vi "Core.vi"(8 "error in (no error)":errorcluster, 11 "TCP in":refnum<class "TCP.lvclass">) -> (0 "error out":errorcluster, 3 "TCP out":refnum<class "TCP.lvclass">)   [LabVIEW 2021, in "TCP.lvclass"]
uses:
  TCP.lvclass
  D:/my_projects/projects/Algorithms/Labview/21/Modbus_v121c/Network Protocol/MB/Modbus Master CR.lvclass
  MB/ctl/MB_TCP_State.ctl
  MB/Modbus Master CR.lvclass/Modbus Master CR.ctl
  MB/Status/Run/Write Run.vi
  MB/Status/write/Write write.vi
  Data Model/Device Data Model.lvclass
  MB/Modbus Master CR.lvclass
panel:
  out "MB_TCP_State":T1=enum."requests"
  in  "write enable":bool=TRUE
  in  "stop":bool
  out "stopped":bool
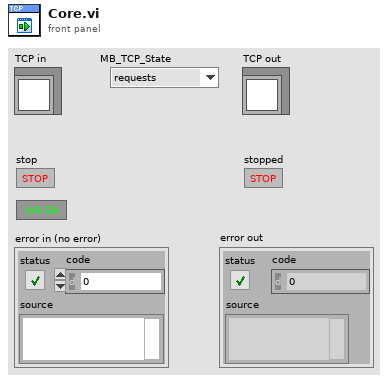
[diagram p1: front panel]
types:
  T1 = typedef "Modbus Master CR.lvclass/MB_TCP_State.ctl" = enum8{"initialization", "redefine", "standby", "ping", "connect", "wait to reconnect", "wait to reset timeout", "configure", "requests", "close connection", "stop"}
  T2 = typedef "Modbus Master CR.lvclass/MB timeouts.ctl" = cluster{"reconn_timeout":i32, "N attempt max":i32, "t_reset_TTL":i32, "period":i32}
  T3 = typedef "Modbus Master CR.lvclass/MB state.ctl" = cluster{"state":T1, "enable":bool, "Run":bool, "write enable":bool, "Write":bool, "connect":bool, "errors":i32}
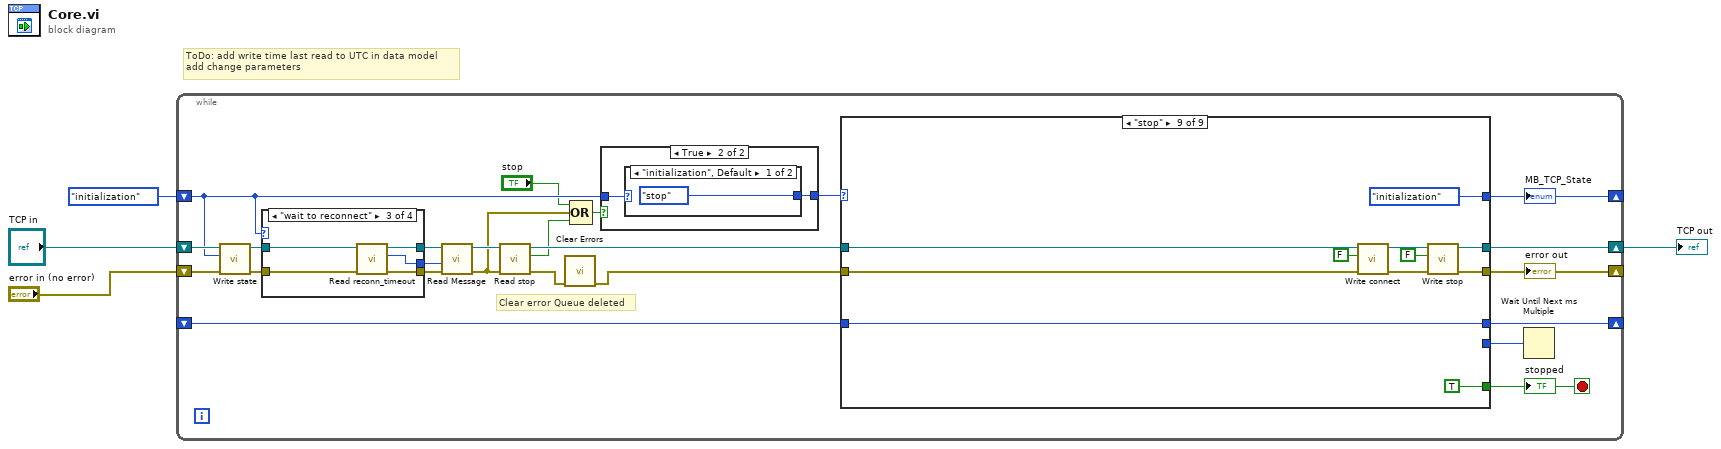
[diagram p0: block diagram]
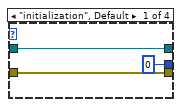
[diagram p2: hidden frame]
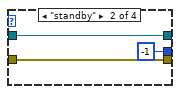
[diagram p3: hidden frame]
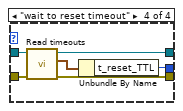
[diagram p4: hidden frame]
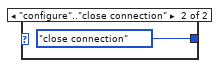
[diagram p6: hidden frame]
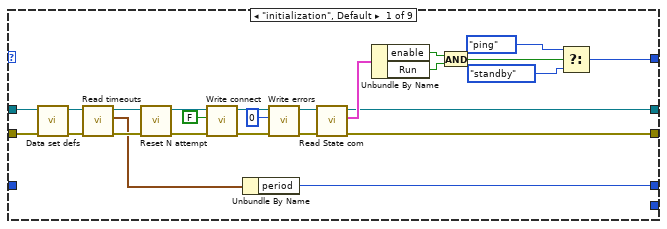
[diagram p7: hidden frame]
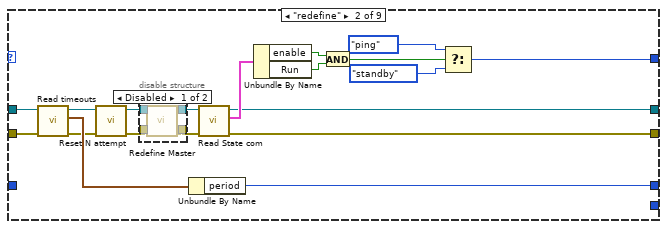
[diagram p8: hidden frame]
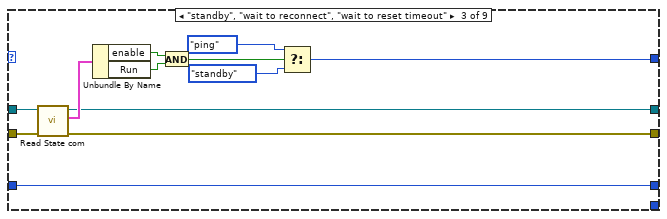
[diagram p10: hidden frame]
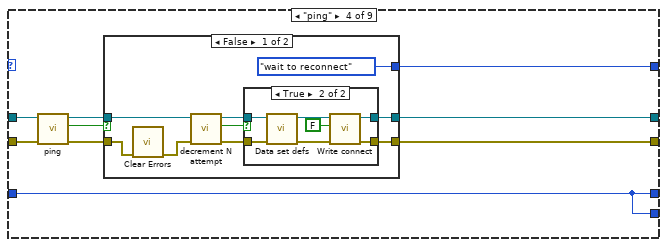
[diagram p11: hidden frame]
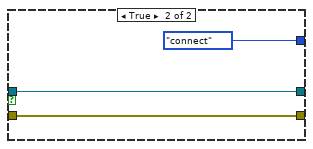
[diagram p13: hidden frame]
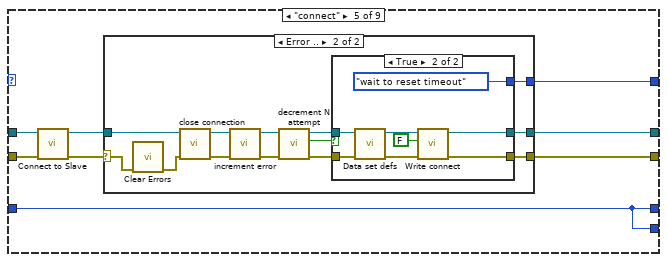
[diagram p14: hidden frame]
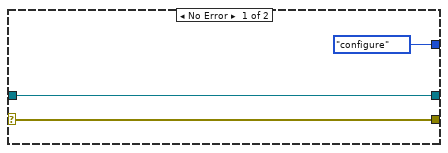
[diagram p15: hidden frame]
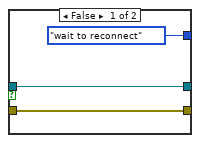
[diagram p16: hidden frame]
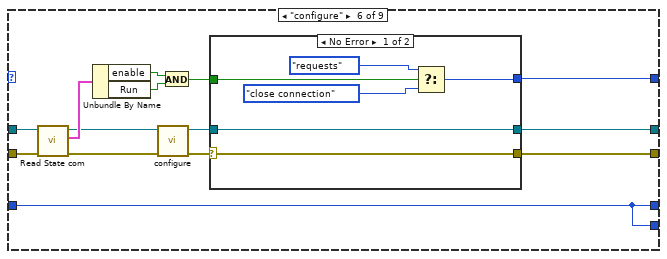
[diagram p17: hidden frame]
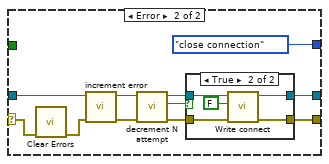
[diagram p18: hidden frame]
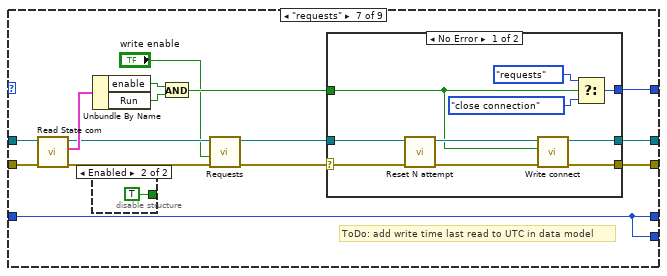
[diagram p20: hidden frame]
diagram:
  # "ToDo: add write time last read to UTC in data model\nadd change parameters"
  n1 = while {
    shift-right: [w25] -> w2
    shift-left: "TCP in" -> [w20]
    shift-right: [w11] -> _
    shift-left: "error in (no error)" -> [w19]
    shift-right: [w27] -> _
    shift-left: _ -> [w28]
    shift-right: [w12] -> _
    shift-left: MB_TCP_State."initialization" ("state") -> [w16]
    stop <- w10 stop-if-true
    # "Clear error Queue deleted"
    n2 = call "Write state.vi"("error in (no error)"=w19, "state"=w16, "MB in"=w20) -> ("error out"=w17:errorcluster, "MB out"=w18:refnum<class "TCP.lvclass">)  [unwired: 7 in]
    n3 = case shown="\"wait to reconnect\"" w16 {
      tunnel: w18 -> [w30 w33 w39 w44]
      tunnel: w17 -> [w29 w32 w38 w43]
      tunnel: [w30 w33 w37 w42] -> w23
      tunnel: [w29 w32 w36 w41] -> w22
      tunnel: [0 ("timeout (0)") -1 ("timeout (0)") w35 w40] -> w21
      frame "initialization", Default {
      }
      frame "standby" {
      }
      frame "wait to reconnect" {
        n4 = call "Read reconn_timeout.vi"("error in (no error)"=w38, "MB_TCP in"=w39) -> ("error out"=w36:errorcluster, "reconn_timeout"=w35:i32, "MB_TCP out"=w37:refnum<class "TCP.lvclass">)  [unwired: 7 in]
      }
      frame "wait to reset timeout" {
        n5 = call "Read timeouts.vi"("error in (no error)"=w43, "MB_TCP in"=w44) -> ("error out"=w41:errorcluster, "MB timeouts"=w45:T2, "MB_TCP out"=w42:refnum<class "TCP.lvclass">)  [unwired: 7 in]
        n6 = Unbundle By Name(w45) -> ("t_reset_TTL"=w40:i32)
      }
    }
    n7 = call "Read Message.vi"("error in (no error)"=w22, "timeout (0)"=w21, "MB in"=w23) -> ("error out"=w8:errorcluster, "MB out"=w14:refnum<class "TCP.lvclass">)  [unwired: 6 in, 1 out]
    n8 = call "Read stop.vi"("error in (no error)"=w8, "MB in"=w14) -> ("error out"=w7:errorcluster, "Stop"=w9:bool, "MB out"=w13:refnum<class "TCP.lvclass">)  [unwired: 7 in]
    n9 = call <vilib>:"Clear Errors.vi"("error in (no error)"=w7) -> ("error out"=w6:errorcluster)  [unwired: 5 in, 1 out]
    n10 = Compound Arithmetic op=OR("stop", w8, w9) -> (w15:bool)
    n11 = case shown="True" w15 {
      tunnel: w16 -> [w46 w48]
      tunnel: [w46 w47] -> w24
      frame False {
      }
      frame True {
        n12 = case shown="\"initialization\", Default" w48 {
          tunnel: [MB_TCP_State."stop" ("MB_TCP_State") MB_TCP_State."close connection" ("MB_TCP_State")] -> w47
          frame "initialization", Default {
          }
          frame "configure".."close connection" {
          }
        }
      }
    }
    n13 = case shown="\"stop\"" w24 {
      tunnel: [_ _ _ _ _ _ _ _ TRUE] -> w10
      tunnel: w13 -> [w73 w91 w105 w117 w146 w182 w219 w276 w283]
      tunnel: [w53 w77 w102 w121 w150 w191 w230 w269 w286] -> w25
      tunnel: w6 -> [w74 w90 w104 w116 w147 w181 w218 w275 w282]
      tunnel: [w51 w92 w101 w120 w149 w190 w229 w261 MB_TCP_State."initialization" ("MB_TCP_State")] -> w12
      tunnel: [w52 w78 w103 w119 w148 w189 w228 w268 w285] -> w11
      tunnel: [w75 w88 w112 w118 w143 w188 w226 w277 w290] -> w27
      tunnel: w28 -> [_ _ w112 w118 w143 w188 w226 w277 w290]
      tunnel: [_ _ _ w118 w143 w188 w226 _ _] -> w26
      frame "initialization", Default {
        n14 = call "Data set defs.vi"("error in (no error)"=w74, "MB_TCP in"=w73) -> ("error out"=w68:errorcluster, "MB_TCP out"=w71:refnum<class "TCP.lvclass">)  [unwired: 8 in]
        n15 = call "Read timeouts.vi"("error in (no error)"=w68, "MB_TCP in"=w71) -> ("error out"=w72:errorcluster, "MB timeouts"=w69:T2, "MB_TCP out"=w70:refnum<class "TCP.lvclass">)  [unwired: 7 in]
        n16 = call "Reset N attempt.vi"("error in (no error)"=w72, "MB_TCP in"=w70) -> ("error out"=w66:errorcluster, "MB_TCP out"=w67:refnum<class "TCP.lvclass">)  [unwired: 8 in]
        n17 = call "Write connect.vi"("error in (no error)"=w66, "connect"=FALSE, "MB in"=w67) -> ("error out"=w64:errorcluster, "MB out"=w63:refnum<class "TCP.lvclass">)  [unwired: 7 in]
        n18 = Unbundle By Name(w69) -> ("period"=w75:i32)
        n19 = call "Write errors.vi"("error in (no error)"=w64, "errors"=0, "MB in"=w63) -> ("error out"=w54:errorcluster, "MB out"=w55:refnum<class "TCP.lvclass">)  [unwired: 7 in]
        n20 = call "Read State com.vi"("error in (no error)"=w54, "MB_TCP in"=w55) -> ("error out"=w52:errorcluster, "State com"=w61:T3, "MB_TCP out"=w53:refnum<class "TCP.lvclass">)  [unwired: 7 in]
        n21 = Unbundle By Name(w61) -> ("enable"=w60:bool, "Run"=w59:bool)
        n22 = And(x=w60, y=w59) -> (x .and. y?=w58:bool)
        n23 = Select(t=MB_TCP_State."ping" ("MB_TCP_State"), s=w58, f=MB_TCP_State."standby" ("MB_TCP_State")) -> (s? t:f=w51:T1)
      }
      frame "redefine" {
        n24 = call "Read timeouts.vi"("error in (no error)"=w90, "MB_TCP in"=w91) -> ("error out"=w87:errorcluster, "MB timeouts"=w89:T2, "MB_TCP out"=w86:refnum<class "TCP.lvclass">)  [unwired: 7 in]
        n25 = call "Reset N attempt.vi"("error in (no error)"=w87, "MB_TCP in"=w86) -> ("error out"=w84:errorcluster, "MB_TCP out"=w85:refnum<class "TCP.lvclass">)  [unwired: 8 in]
        n26 = disable-structure shown="Disabled" {
          disable-tunnel: w85 -> [w98 w100]
          disable-tunnel: w84 -> [w97 w99]
          disable-tunnel: [w96 w100] -> w80
          disable-tunnel: [w95 w99] -> w79
          frame Disabled {
            n27 = call "Redefine Master.vi"("error in (no error)"=w97, "MB_TCP in"=w98) -> ("error out"=w95:errorcluster, "MB_TCP out"=w96:refnum<class "TCP.lvclass">)  [unwired: 8 in]
          }
          frame Enabled {
          }
        }
        n28 = Unbundle By Name(w89) -> ("period"=w88:i32)
        n29 = call "Read State com.vi"("error in (no error)"=w79, "MB_TCP in"=w80) -> ("error out"=w78:errorcluster, "State com"=w83:T3, "MB_TCP out"=w77:refnum<class "TCP.lvclass">)  [unwired: 7 in]
        n30 = Unbundle By Name(w83) -> ("enable"=w82:bool, "Run"=w81:bool)
        n31 = And(x=w82, y=w81) -> (x .and. y?=w76:bool)
        n32 = Select(t=MB_TCP_State."ping" ("MB_TCP_State"), s=w76, f=MB_TCP_State."standby" ("MB_TCP_State")) -> (s? t:f=w92:T1)
      }
      frame "standby", "wait to reconnect", "wait to reset timeout" {
        n33 = call "Read State com.vi"("error in (no error)"=w104, "MB_TCP in"=w105) -> ("error out"=w103:errorcluster, "State com"=w111:T3, "MB_TCP out"=w102:refnum<class "TCP.lvclass">)  [unwired: 7 in]
        n34 = Unbundle By Name(w111) -> ("enable"=w110:bool, "Run"=w109:bool)
        n35 = And(x=w110, y=w109) -> (x .and. y?=w108:bool)
        n36 = Select(t=MB_TCP_State."ping" ("MB_TCP_State"), s=w108, f=MB_TCP_State."standby" ("MB_TCP_State")) -> (s? t:f=w101:T1)
      }
      frame "ping" {
        n37 = call-dynamic "ping.vi"("error in (no error)"=w116, "TCP in"=w117) -> ("error out"=w113:errorcluster, "Ping OK"=w114:bool, "TCP out"=w115:refnum<class "TCP.lvclass">)  [unwired: 7 in]
        n38 = case shown="False" w114 {
          tunnel: w115 -> [w124 w142]
          tunnel: [MB_TCP_State."wait to reconnect" ("MB_TCP_State") MB_TCP_State."connect" ("MB_TCP_State")] -> w120
          tunnel: [w129 w142] -> w121
          tunnel: [w128 w140] -> w119
          tunnel: w113 -> [w125 w140]
          frame False {
            n39 = call <vilib>:"Clear Errors.vi"("error in (no error)"=w125) -> ("error out"=w123:errorcluster)  [unwired: 5 in, 1 out]
            n40 = call "decrement N attempt.vi"("error in (no error)"=w123, "MB_TCP in"=w124) -> ("error out"=w126:errorcluster, "=0"=w130:bool, "MB_TCP out"=w127:refnum<class "TCP.lvclass">)  [unwired: 7 in]
            n41 = case shown="True" w130 {
              tunnel: w127 -> [w132 w139]
              tunnel: [w132 w136] -> w129
              tunnel: w126 -> [w131 w138]
              tunnel: [w131 w133] -> w128
              frame False {
              }
              frame True {
                n42 = call "Data set defs.vi"("error in (no error)"=w138, "MB_TCP in"=w139) -> ("error out"=w134:errorcluster, "MB_TCP out"=w137:refnum<class "TCP.lvclass">)  [unwired: 8 in]
                n43 = call "Write connect.vi"("error in (no error)"=w134, "connect"=FALSE, "MB in"=w137) -> ("error out"=w133:errorcluster, "MB out"=w136:refnum<class "TCP.lvclass">)  [unwired: 7 in]
              }
            }
          }
          frame True {
          }
        }
      }
      frame "connect" {
        n44 = call-dynamic "Connect to Slave.vi"("error in (no error)"=w147, "network master in"=w146) -> ("error out"=w144:errorcluster, "network master out"=w145:refnum<class "TCP.lvclass">)  [unwired: 8 in]
        n45 = case shown="Error .." w144 {
          selector: w144 -> [w151 w158]
          tunnel: w145 -> [w152 w159]
          tunnel: [MB_TCP_State."configure" ("MB_TCP_State") w164] -> w149
          tunnel: [w152 w163] -> w150
          tunnel: [w151 w162] -> w148
          frame No Error {
          }
          frame Error {
            n46 = call <vilib>:"Clear Errors.vi"("error in (no error)"=w158) -> ("error out"=w157:errorcluster)  [unwired: 5 in, 1 out]
            n47 = call-dynamic "close connection.vi"("error in (no error)"=w157, "MB in"=w159) -> ("error out"=w160:errorcluster, "MB out"=w161:refnum<class "TCP.lvclass">)  [unwired: 8 in]
            n48 = call "increment error.vi"("error in (no error)"=w160, "MB_TCP in"=w161) -> ("error out"=w156:errorcluster, "MB_TCP out"=w166:refnum<class "TCP.lvclass">)  [unwired: 7 in, 1 out]
            n49 = call "decrement N attempt.vi"("error in (no error)"=w156, "MB_TCP in"=w166) -> ("error out"=w154:errorcluster, "=0"=w165:bool, "MB_TCP out"=w155:refnum<class "TCP.lvclass">)  [unwired: 7 in]
            n50 = case shown="True" w165 {
              tunnel: [MB_TCP_State."wait to reconnect" ("MB_TCP_State") MB_TCP_State."wait to reset timeout" ("MB_TCP_State")] -> w164
              tunnel: w155 -> [w168 w176]
              tunnel: [w168 w173] -> w163
              tunnel: w154 -> [w167 w175]
              tunnel: [w167 w170] -> w162
              frame False {
              }
              frame True {
                n51 = call "Data set defs.vi"("error in (no error)"=w175, "MB_TCP in"=w176) -> ("error out"=w171:errorcluster, "MB_TCP out"=w174:refnum<class "TCP.lvclass">)  [unwired: 8 in]
                n52 = call "Write connect.vi"("error in (no error)"=w171, "connect"=FALSE, "MB in"=w174) -> ("error out"=w170:errorcluster, "MB out"=w173:refnum<class "TCP.lvclass">)  [unwired: 7 in]
              }
            }
          }
        }
      }
      frame "configure" {
        n53 = call "Read State com.vi"("error in (no error)"=w181, "MB_TCP in"=w182) -> ("error out"=w180:errorcluster, "State com"=w185:T3, "MB_TCP out"=w179:refnum<class "TCP.lvclass">)  [unwired: 7 in]
        n54 = Unbundle By Name(w185) -> ("enable"=w184:bool, "Run"=w183:bool)
        n55 = call-dynamic "configure.vi"("error in (no error)"=w180, "MB_TCP in"=w179) -> ("error out"=w186:errorcluster, "MB_TCP out"=w187:refnum<class "TCP.lvclass">)  [unwired: 8 in]
        n56 = And(x=w184, y=w183) -> (x .and. y?=w178:bool)
        n57 = case shown="No Error" w186 {
          selector: w186 -> [w193 w207]
          tunnel: [w197 MB_TCP_State."close connection" ("MB_TCP_State")] -> w190
          tunnel: [w193 w200] -> w189
          tunnel: w187 -> [w194 w199]
          tunnel: [w194 w201] -> w191
          tunnel: w178 -> [w192 _]
          frame No Error {
            n58 = Select(t=MB_TCP_State."requests" ("MB_TCP_State"), s=w192, f=MB_TCP_State."close connection" ("MB_TCP_State")) -> (s? t:f=w197:T1)
          }
          frame Error {
            n59 = call <vilib>:"Clear Errors.vi"("error in (no error)"=w207) -> ("error out"=w198:errorcluster)  [unwired: 5 in, 1 out]
            n60 = call "increment error.vi"("error in (no error)"=w198, "MB_TCP in"=w199) -> ("error out"=w203:errorcluster, "MB_TCP out"=w202:refnum<class "TCP.lvclass">)  [unwired: 7 in, 1 out]
            n61 = call "decrement N attempt.vi"("error in (no error)"=w203, "MB_TCP in"=w202) -> ("error out"=w204:errorcluster, "=0"=w206:bool, "MB_TCP out"=w205:refnum<class "TCP.lvclass">)  [unwired: 7 in]
            n62 = case shown="True" w206 {
              tunnel: w205 -> [w210 w215]
              tunnel: [w210 w214] -> w201
              tunnel: w204 -> [w209 w213]
              tunnel: [w209 w211] -> w200
              frame False {
              }
              frame True {
                n63 = call "Write connect.vi"("error in (no error)"=w213, "connect"=FALSE, "MB in"=w215) -> ("error out"=w211:errorcluster, "MB out"=w214:refnum<class "TCP.lvclass">)  [unwired: 7 in]
              }
            }
          }
        }
      }
      frame "requests" {
        # "ToDo: add write time last read to UTC in data model"
        n64 = call "Read State com.vi"("error in (no error)"=w218, "MB_TCP in"=w219) -> ("error out"=w220:errorcluster, "State com"=w224:T3, "MB_TCP out"=w221:refnum<class "TCP.lvclass">)  [unwired: 7 in]
        n65 = Unbundle By Name(w224) -> ("enable"=w223:bool, "Run"=w222:bool)
        n66 = disable-structure shown="Enabled" {
          disable-tunnel: [w231 TRUE] -> _
          frame Disabled {
            n67 = Equal?() -> (x = y?=w231:bool)  [unwired: 2 in]
          }
          frame Enabled {
          }
        }
        n68 = And(x=w223, y=w222) -> (x .and. y?=w217:bool)
        n69 = call-dynamic "Requests.vi"("error in (no error)"=w220, "write enable"="write enable", "TCP in"=w221) -> ("error out"=w225:errorcluster, "TCP out"=w227:refnum<class "TCP.lvclass">)  [unwired: 7 in]
        n70 = case shown="No Error" w225 {
          selector: w225 -> [w238 w253]
          tunnel: [w242 MB_TCP_State."close connection" ("MB_TCP_State")] -> w229
          tunnel: w217 -> [w235 _]
          tunnel: [w233 w249] -> w228
          tunnel: w227 -> [w239 w246]
          tunnel: [w236 w250] -> w230
          frame No Error {
            n71 = call "Reset N attempt.vi"("error in (no error)"=w238, "MB_TCP in"=w239) -> ("error out"=w234:errorcluster, "MB_TCP out"=w237:refnum<class "TCP.lvclass">)  [unwired: 8 in]
            n72 = call "Write connect.vi"("error in (no error)"=w234, "connect"=w235, "MB in"=w237) -> ("error out"=w233:errorcluster, "MB out"=w236:refnum<class "TCP.lvclass">)  [unwired: 7 in]
            n73 = Select(t=MB_TCP_State."requests" ("MB_TCP_State"), s=w235, f=MB_TCP_State."close connection" ("MB_TCP_State")) -> (s? t:f=w242:T1)
          }
          frame Error {
            # "clear read error"
            n74 = call <vilib>:"Clear Errors.vi"("error in (no error)"=w253) -> ("error out"=w245:errorcluster)  [unwired: 5 in, 1 out]
            n75 = call "increment error.vi"("error in (no error)"=w245, "MB_TCP in"=w246) -> ("error out"=w247:errorcluster, "MB_TCP out"=w252:refnum<class "TCP.lvclass">)  [unwired: 7 in, 1 out]
            n76 = call "decrement N attempt.vi"("error in (no error)"=w247, "MB_TCP in"=w252) -> ("error out"=w248:errorcluster, "=0"=w244:bool, "MB_TCP out"=w251:refnum<class "TCP.lvclass">)  [unwired: 7 in]
            n77 = case shown="True" w244 {
              tunnel: w251 -> [w255 w260]
              tunnel: [w255 w259] -> w250
              tunnel: w248 -> [w254 w258]
              tunnel: [w254 w256] -> w249
              frame False {
              }
              frame True {
                n78 = call "Write connect.vi"("error in (no error)"=w258, "connect"=FALSE, "MB in"=w260) -> ("error out"=w256:errorcluster, "MB out"=w259:refnum<class "TCP.lvclass">)  [unwired: 7 in]
              }
            }
          }
        }
      }
      frame "close connection" {
        n79 = call-dynamic "close connection.vi"("error in (no error)"=w275, "MB in"=w276) -> ("error out"=w270:errorcluster, "MB out"=w271:refnum<class "TCP.lvclass">)  [unwired: 8 in]
        n80 = call "Read State com.vi"("error in (no error)"=w270, "MB_TCP in"=w271) -> ("error out"=w268:errorcluster, "State com"=w274:T3, "MB_TCP out"=w269:refnum<class "TCP.lvclass">)  [unwired: 7 in]
        n81 = Unbundle By Name(w274) -> ("enable"=w273:bool, "Run"=w272:bool)
        n82 = disable-structure shown="Enabled" {
          disable-tunnel: [w278 TRUE] -> w262
          frame Disabled {
            n83 = Equal?() -> (x = y?=w278:bool)  [unwired: 2 in]
          }
          frame Enabled {
          }
        }
        n84 = And(x=w273, y=w272) -> (x .and. y?=w263:bool)
        n85 = Select(t=MB_TCP_State."wait to reconnect" ("MB_TCP_State"), s=w262, f=MB_TCP_State."redefine" ("MB_TCP_State")) -> (s? t:f=w265:T1)
        n86 = Select(t=w265, s=w263, f=MB_TCP_State."standby" ("MB_TCP_State")) -> (s? t:f=w261:T1)
      }
      frame "stop" {
        n87 = call "Write connect.vi"("error in (no error)"=w282, "connect"=FALSE, "MB in"=w283) -> ("error out"=w281:errorcluster, "MB out"=w284:refnum<class "TCP.lvclass">)  [unwired: 7 in]
        n88 = call "Write stop.vi"("error in (no error)"=w281, "Stop"=FALSE, "MB in"=w284) -> ("error out"=w285:errorcluster, "MB out"=w286:refnum<class "TCP.lvclass">)  [unwired: 7 in]
      }
    }
    "stopped" <- w10
    "error out" <- w11
    "MB_TCP_State" <- w12
    n89 = Wait Until Next ms Multiple(millisecond multiple=w26) -> ()  [unwired: 1 out]
  }
  "TCP out" <- w2
